vi "Get Head Info.vi"(8 "error in":errorcluster, 9 "Head Channel":i16, 10 "Pulsar Handle":i16, 11 "OphirFastX (in)":refnum<k7>) -> (0 "error out":errorcluster, 3 "OphirFastX (out)":refnum<k7>, 5 "Head Info":string)   [LabVIEW 2009]
panel:
  # "Guillaume Plateau - yguig2@yahoo.fr"
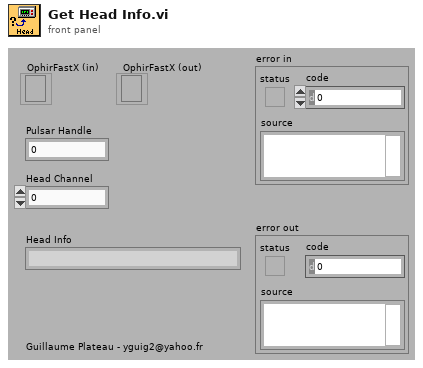
[diagram p1: front panel]
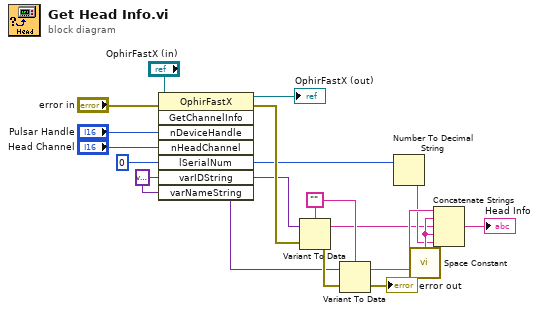
[diagram p0: block diagram]
diagram:
  w8 = variant ("varIDString")
  w10 = ""
  n1 = invoke class="OphirFastX" method="GetChannelInfo"(reference="OphirFastX (in)", error in="error in", "nDeviceHandle"="Pulsar Handle", "nHeadChannel"="Head Channel", "lSerialNum"=0, "varIDString"=w8, "varNameString"=w8) -> (reference out=→"OphirFastX (out)":refnum<k7>, error out=w16:errorcluster, "lSerialNum"=w5:i32, "varIDString"=w11:variant, "varNameString"=w9:variant)  [unwired: 1 in, 3 out]
  n2 = Variant To Data(error in=w16, Variant=w11, type=w10) -> (error out=w15:errorcluster, data=w4:string)
  n3 = Variant To Data(error in=w15, Variant=w9, type=w10) -> (error out=→"error out":errorcluster, data=w13:string)
  n4 = Number To Decimal String(number=w5) -> (decimal integer string=w12:string)  [unwired: 1 in]
  n5 = call <vilib>:"Space Constant.vi"() -> ("String"=w14:string)
  n6 = Concatenate Strings(w13, w14, w4, w14, w12) -> (→"Head Info":string)
